vi "AddTextForNotifier.vi"(0 "error in (no error)":errorcluster, 3 "Text in":string, 4 "Command":string) -> (5 "Text out":string)   [LabVIEW 2012]
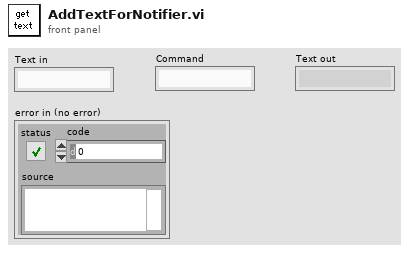
[diagram p1: front panel]
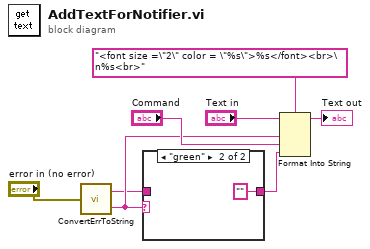
[diagram p0: block diagram]
diagram:
  n1 = call <userlib>:"ConvertErrToString.vi"("error in (no error)"="error in (no error)") -> ("String"=w1:string, "color"=w3:string)
  n2 = case shown="\"green\"" w3 {
    tunnel: [w9 "" ("String")] -> w2
    tunnel: w1 -> [w9 _]
    frame Default {
    }
    frame "green" {
    }
  }
  n3 = Format Into String(format string="<font size =\"2\" color = \"%s\">%s</font><br>\n%s<br>", initial string="Text in", w3, "Command", w2) -> (resulting string=→"Text out":string)  [unwired: 1 in, 1 out]
